vi "GlobalVars.vi"() -> ()   [LabVIEW 2019]
panel:
  out "GlobalTime":dbl
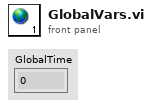
[diagram p1: front panel]
diagram:
